vi "RunIconEditor.vi"(8 "error in (no error)":errorcluster, 11 "Library Refnum in":refnum<vi>) -> (0 "error out":errorcluster, 1 "Canceled?":bool, 2 "Icon out":refnum<class "Icon.lvclass">, 3 "Library Refnum out":refnum<vi>)   [LabVIEW 2014, in "BasicClassDocumentation.lvlib" / "BasicClassDocumentation.lvclass"]
uses:
  BasicClassDocumentation.lvclass
  <vilib>/LabVIEW Icon API/lv_icon/Classes/Icon/Icon.lvclass
  <vilib>/LabVIEW Icon API/LabVIEW Icon API.lvlib
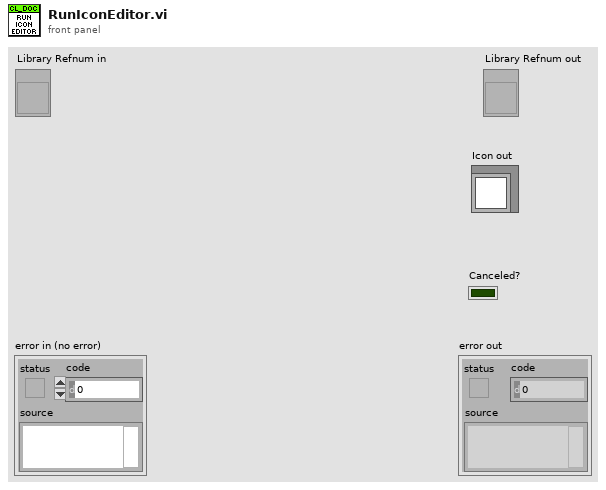
[diagram p1: front panel]
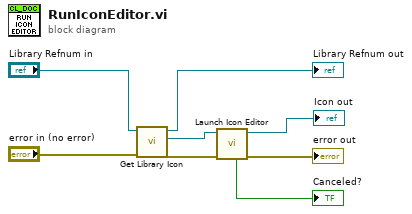
[diagram p0: block diagram]
diagram:
  n1 = call <vilib>:"Get Library Icon.vi"("error in (no error)"="error in (no error)", "Library Refnum in"="Library Refnum in") -> ("error out"=w7:errorcluster, "Icon"=w8:refnum<class "Icon.lvclass">, "Library Refnum out"=→"Library Refnum out":refnum<vi>)  [unwired: 7 in]
  n2 = call <vilib>:"Launch Icon Editor.vi"("error in (no error)"=w7, "Icon in"=w8) -> ("error out"=→"error out":errorcluster, "Icon out"=→"Icon out":refnum<class "Icon.lvclass">, "Canceled?"=→"Canceled?":bool)  [unwired: 7 in]
